vi "H5Oopen.vi"(5 "lapl_id":T1, 6 "error in (no error)":errorcluster, 8 "Name":string, 9 "Location Ref":T1) -> (0 "error out":errorcluster, 2 "Object Ref":T1, 3 "Location Ref out":T1)   [LabVIEW 2017]
doc: "Opens an object in an HDF5 file by location identifier and path name."
uses:
  <vilib>/UPVI/lvhdf5/library.llb/HDF5 Ref.ctl
  <vilib>/UPVI/lvhdf5/hdf5.dll
panel:
  # "LVHDF5 Toolkit\nCopyright (c) 2005-2013 by Jason D. Sommerville\nCopyright (c) 2014-2015 by UPVI, LLC.\n\nThis use and distribution of this file is governed by the terms found in \nLICENSE.txt distributed with this toolkit and installed at\n <user.lib>\\_lvhdf5\\LICENSE.txt"
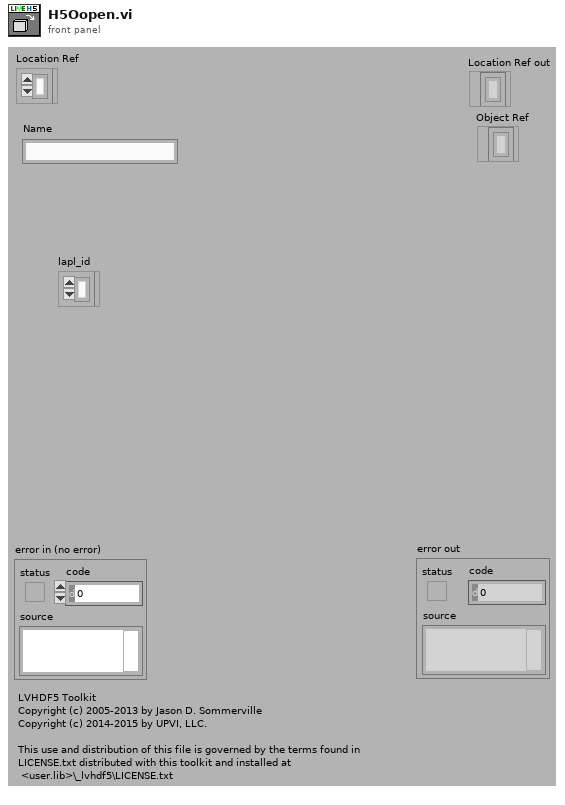
[diagram p1: front panel]
types:
  T1 = typedef "HDF5 Ref.ctl" = refnum<k1>
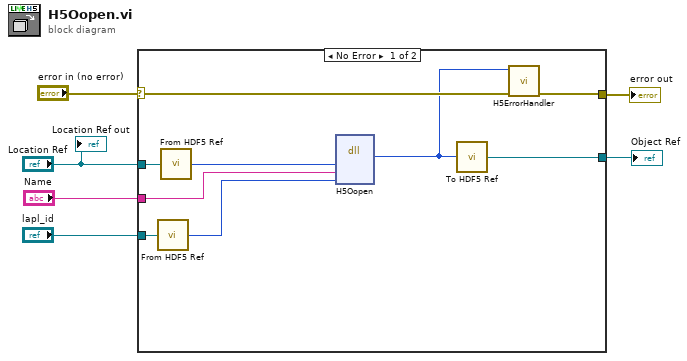
[diagram p0: block diagram]
diagram:
  n1 = case shown="No Error" "error in (no error)" {
    selector: "error in (no error)" -> [w15 w16]
    tunnel: [w14 w16] -> w5
    tunnel: "Location Ref" -> [w13 _]
    tunnel: "Name" -> [w11 _]
    tunnel: "lapl_id" -> [w10 _]
    tunnel: [w7 _] -> w1
    frame No Error {
      n2 = call <vilib>:"From HDF5 Ref.vi"("HDF5 Ref"=w10) -> ("I32"=w9:i32)
      n3 = call <vilib>:"From HDF5 Ref.vi"("HDF5 Ref"=w13) -> ("I32"=w12:i32)
      n4 = dll-call lib="C:/Program Files/National Instruments/LabVIEW 2017/vi.lib/UPVI/lvhdf5/hdf5.dll" fn="H5Oopen" label="H5Oget_info"("loc_id"=w12, "name"=w11, "lapl_id"=w9) -> ("return type"=w8:i32)  [unwired: 6 in, 2 out]
      n5 = call <vilib>:"To HDF5 Ref.vi"("I32"=w8) -> ("HDF5 Ref"=w7:T1)
      n6 = call <vilib>:"H5ErrorHandler.vi"("error in (no error)"=w15, "herr_t"=w8) -> ("error out"=w14:errorcluster)  [unwired: 3 in, 4 out]
    }
    frame Error {
    }
  }
  "error out" <- w5
  "Object Ref" <- w1
  "Location Ref out" <- "Location Ref"
